vi "testDataPass_v2,0_global1.vi"() -> ()   [LabVIEW 2014]
panel:
  in  "arrTF":bool[](array[boolean])
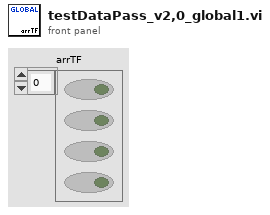
[diagram p1: front panel]
diagram:
